vi "PH_PowerUnit_BaseClass.check Waiting state.vi"(0 "i ref in":refnum<vi>, 5 "error in (no error)":errorcluster) -> (14 "i ref out":refnum<vi>, 19 "error out":errorcluster)   [LabVIEW 2014, in "PH_PowerUnit_BaseClass.lvlib"]
doc: "This VI calculates the state of the waiting time: if the waiting time is over, \"true\" is indicated. At the waiting time \"0\" appears at \"Waiting Time (s)\" in this case. Otherwise the remaining waiting is indicated in seconds. If an \"9999\" appears, an error occured by checking the waiting time.\n\n\"Required Device(s) off?\" is true if at least one device is even not switched on."
uses:
  PH_PowerUnit_BaseClass.lvlib
  CSlibraries-extern/DimLVEvent/LVDimInterface/LVDimInterface.lvlib
  PH_Common/PH_Common.lvlib
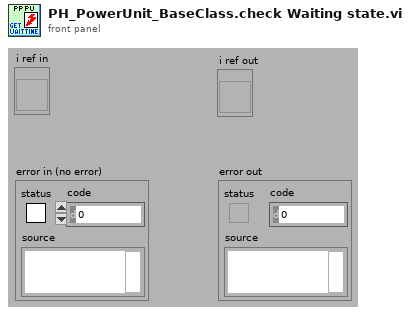
[diagram p1: front panel]
types:
  T1 = typedef "PH_PowerUnit_BaseClass.lvlib/PH_PowerUnit_BaseClass.i attribute.ctl" = cluster{"Constructor finished":bool, "PU":cluster{"In use":bool, "Service ID in use":i32, "GUI Ref":refnum<vi>}, "Enabling":cluster{"State":T2, "GUI Ref":refnum<vi>}, "Timing":cluster{"Last Shot":dbl, "Time between Shots [Sec]":dbl, "Waiting Time over?":bool, "Service ID Waiting Time":i32, "GUI Ref":refnum<vi>, "Instance":cluster{"Status":T3, "linked?":bool, "GUI Ref":refnum<vi>}}, "Sequencer":cluster{"SM State":string, "GUI Ref":refnum<vi>, "linked":bool}, "Subscribed Trendmssgs":cluster{"Tagname":string, "Status":T3, "linked?":bool, "Shot Condition":T3, "GUI Ref":refnum<vi>}[], "PP PU":T4, "Default Voltage (V)":dbl, "GUI Refs":T5, "PSDB data":cluster{"Shot Voltage [V]":dbl, "State TO SM":T6, "Write 2 early":bool}, "State TO SM":T6}
  T2 = typedef "PH_SystemInformation.lvlib/PH_SystemInformationEnabling State.ctl" = i32
  T3 = typedef "PH_StatusHandler.lvlib/PH_StatusHandler.Status.ctl" = i16
  T4 = typedef "PH_PP_Common.lvlib/PH_PP_Common.PUs.ctl" = enum16{"no Info", "PA-19mm-1", "PA-19mm-2", "PA-45mm-PILC", "PA-45mm-MAIN", "MA-PU-1", "MA-PU-2", "MA-PU-3", "MA-PU-4", "MA-PU-5", "MA-PU-6", "MA-FR", "MA-PILC", "PA-45mm-DP"}
  T5 = typedef "PH_PowerUnit_BaseClass.lvlib/PH_PowerUnit_BaseClass.GUI Refs.ctl" = cluster{"Delete Inst":refnum<vi>, "State TO SM":refnum<vi>, "State SM":refnum<vi>, "Fire":refnum<vi>}
  T6 = typedef "PH_PowerUnit_BaseClass.lvlib/PH_PowerUnit_BaseClass.SM States.ctl" = enum16{".", "Stand by", "Switch PU on", "Configure", "Set Default Voltage", "Set STANDBY", "Set READY", "Wait for Shot Cmd", "Open Dump Rods", "Open Ross Relais", "Close Ross Relais", "Switch PSU on", "Switch PSU off", "Charge", "Switch GD Channel on", "Close Dump Rods", "Rods-TO", "RR-TO", "PSU-TO", "Trigger-TO"}
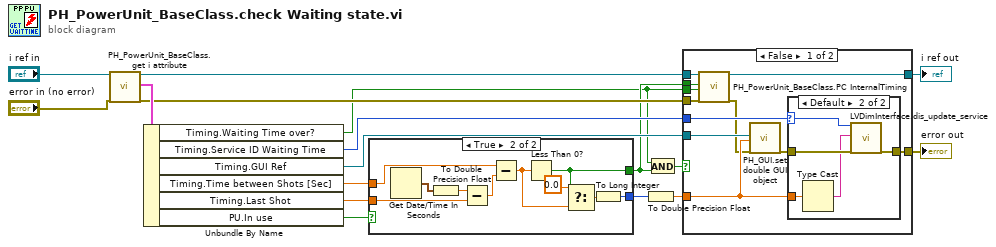
[diagram p0: block diagram]
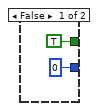
[diagram p2: hidden frame]
diagram:
  n1 = call "PH_PowerUnit_BaseClass.get i attribute.vi"("i ref in"="i ref in", "error in (no error)"="error in (no error)") -> ("i ref out"=w11:refnum<vi>, "i attribute"=w14:T1, "error out"=w10:errorcluster)  [unwired: 15 in]
  n2 = Unbundle By Name(w14) -> ("Timing.Waiting Time over?"=w2:bool, "Timing.Service ID Waiting Time"=w7:i32, "Timing.GUI Ref"=w8:refnum<vi>, "Timing.Time between Shots [Sec]"=w15:dbl, "Timing.Last Shot"=w9:dbl, "PU.In use"=w1:bool)
  n3 = case shown="True" w1 {
    tunnel: w15 -> [_ w27]
    tunnel: w9 -> [_ w25]
    tunnel: [TRUE w24] -> w3
    tunnel: [0 w20] -> w6
    frame False {
    }
    frame True {
      n4 = Get Date/Time In Seconds() -> (seconds since 1Jan1904=w29:timestamp)
      n5 = To Double Precision Float(number=w29) -> (double precision float=w28:dbl)
      n6 = Subtract(x=w28, y=w25) -> (x-y=w26:dbl)
      n7 = Subtract(x=w27, y=w26) -> (x-y=w22:dbl)
      n8 = Less Than 0?(x=w22) -> (x < 0?=w24:bool)
      n9 = Select(t=0.0, s=w24, f=w22) -> (s? t:f=w21:dbl)
      n10 = To Long Integer(number=w21) -> (32bit integer=w20:i32)
    }
  }
  n11 = To Double Precision Float(number=w6) -> (double precision float=w5:dbl)
  n12 = And(x=w2, y=w3) -> (x .and. y?=w4:bool)
  n13 = case shown="False" w4 {
    tunnel: w10 -> [w32 w47]
    tunnel: [w37 w47] -> w12
    tunnel: w11 -> [w40 w48]
    tunnel: [w39 w48] -> w13
    tunnel: w3 -> [w38 _]
    tunnel: w5 -> [w35 _]
    tunnel: w7 -> [w36 _]
    tunnel: w8 -> [w34 _]
    tunnel: w2 -> [w33 _]
    frame False {
      n14 = call "PH_PowerUnit_BaseClass.PC InternalTiming.vi"("i ref in"=w40, "Waiting Time over? new"=w38, "Waiting Time over? old"=w33, "error in (no error)"=w32) -> ("i ref out"=w39:refnum<vi>, "error out"=w31:errorcluster)  [unwired: 14 in]
      n15 = call "PH_GUI.set double GUI object.vi"("GUI object Ref"=w34, "value"=w35, "error in (no error)"=w31) -> ("error out"=w30:errorcluster)  [unwired: 16 in]
      n16 = case shown="Default" w36 {
        selector: w36 -> [_ w44]
        tunnel: [w41 w45] -> w37
        tunnel: w30 -> [w41 w46]
        tunnel: w35 -> [_ w42]
        frame -1 {
        }
        frame Default {
          n17 = Type Cast(x=w42) -> (*(type *) &x=w43:string)  [unwired: 1 in]
          n18 = call "LVDimInterface.dis_update_service.vi"("my_serviceID"=w44, "data"=w43, "error in (no error)"=w46) -> ("error out"=w45:errorcluster)  [unwired: 14 in, 2 out]
        }
      }
    }
    frame True {
    }
  }
  "i ref out" <- w13
  "error out" <- w12
